vi "CreatePublicEvents.vi"(8 "error in (no error)":errorcluster, 11 "SMO":refnum<class "SMO.lvclass">) -> (0 "error out":errorcluster, 3 "SMO out":refnum<class "SMO.lvclass">)   [LabVIEW 2019, in "SMO.lvclass"]
doc: "JKI State Machine Objects (SMO) 1.3.0.56\nJKI - JKI\nCopyright (c) 2017, JKI"
uses:
  SMO.lvclass
  Typedefs/SMOState --Enum.ctl
  Typedefs/Reserve State--Enum.ctl
  SMO.lvclass/SMO.ctl
panel:
  # "For instructions on how to use the JKI State Machine Objects, examples and video tutorials, visit:\nhttp://jki.net/state-machine-objects/\n\nJKI State Machine Objects™\nhttp://jki.net/state-machine-objects/\nCopyright (C) 2005-2015, JKI <info@jki.net>\nALL RIGHTS RESERVED"
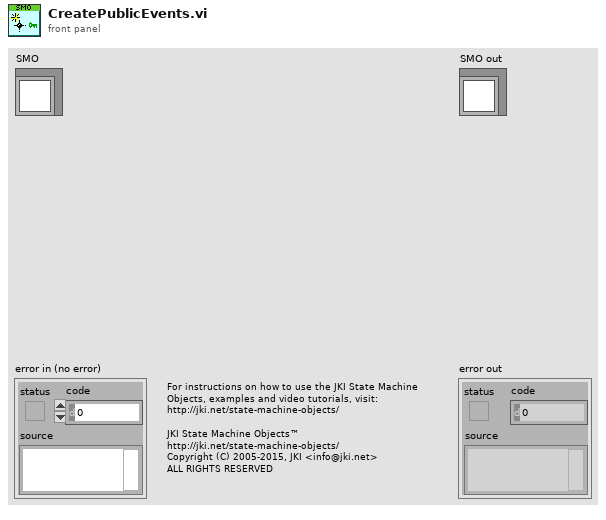
[diagram p1: front panel]
types:
  T1 = typedef "SMO.lvclass/Reserve State--Enum.ctl" = enum16{"Unreserved", "Reserved", "Self-locked"}
  T2 = typedef "SMO.lvclass/SMOState --Enum.ctl" = enum16{"unknown", "Created", "Started", "Stopped"}
  T3 = cluster{"error":refnum<user-event>, "SMO State":refnum<user-event>, "Reserve State":refnum<user-event>}
  T4 = typedef "SMO.lvclass/PrivateData--Ref.ctl" = refnum<data-value>
  T5 = typedef "SMO.lvclass/PrivateData--Cluster.ctl" = cluster{"Parent Call":T6, "Registered Processes":T7[], "Sync Notifier":refnum<notifier>, "Process Error Notifier":refnum<notifier>, "Protected Events":T8, "Public Events":T9, "SMO State":T2, "[Dependencies]":T10[], "[Attributes]":refnum<class "Attribute.lvclass">[], "Launcher Close":refnum<notifier>, "Caller Watchdog":refnum<queue>, "Accessibility":T11, "NbStaticDependencies":u32}
  T6 = typedef "SMO.lvclass/Parent Call--Enum.ctl" = enum16{"Allows parent to run", "Does not request parent to run"}
  T7 = typedef "SMO.lvclass/RegisteredProcessData--Cluster.ctl" = cluster{"Name":string, "Static VI Ref":refnum<vi>, "Running":bool, "NotifierRef":u32}
  T8 = typedef "SMO.lvclass/Protected Events.ctl" = cluster{"StopProcesses":refnum<user-event>, "AbortProcesses":refnum<user-event>, "Config Changed":refnum<user-event>, "Dependency":refnum<user-event>}
  T9 = typedef "SMO.lvclass/Public Events.ctl" = cluster{"Error":refnum<user-event>, "State":refnum<user-event>, "Reserve State":refnum<user-event>}
  T10 = typedef "SMO.lvclass/SMO Dependency--Cluster.ctl" = cluster{"Dependency":refnum<class "SMO.lvclass">, "Level":string}
  T11 = typedef "SMO.lvclass/Accessibility--Cluster.ctl" = cluster{"Lock Key":string, "Reserve State":T1}
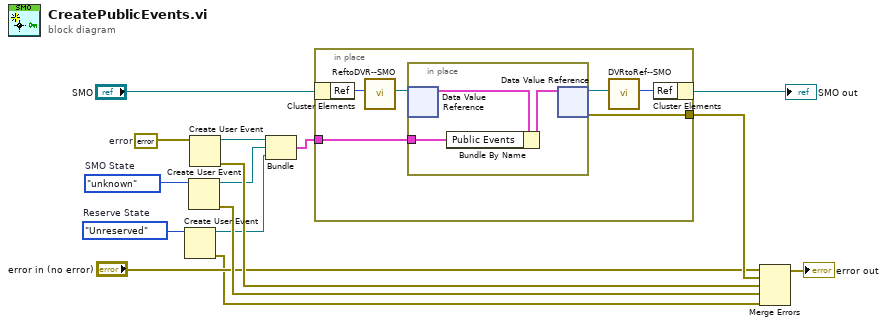
[diagram p0: block diagram]
diagram:
  w2 = Reserve_State--Enum."Unreserved"  # Reserve State
  w7 = SMOState_--Enum."unknown"  # SMO State
  w9 = errorcluster {"status"=FALSE, "code"=0, "source"=""}  # error
  n1 = Create User Event(user event datatype=w2) -> (user event=w1:refnum<user-event>, error out=w3:errorcluster)  [unwired: 1 in]
  n2 = Create User Event(user event datatype=w7) -> (user event=w6:refnum<user-event>, error out=w5:errorcluster)  [unwired: 1 in]
  n3 = Create User Event(user event datatype=w9) -> (user event=w10:refnum<user-event>, error out=w8:errorcluster)  [unwired: 1 in]
  n4 = Bundle("error"=w10, "SMO State"=w6, "Reserve State"=w1) -> (w11:T3)  [unwired: 1 in]
  n5 = in-place {
    in-place-border: w11 -> [w21]
    in-place-border: [w20] -> w12
    n6 = in-place-cluster #1("SMO") -> ("Ref"=w19:u32)
    n7 = call "ReftoDVR--SMO.vi"("Ref"=w19) -> ("Ref"=w18:T4)  [unwired: 10 in]
    n8 = in-place {
      in-place-border: w21 -> [w22]
      n9 = in-place-dvr #2(w18) -> (w24:T5)  [unwired: 1 out]
      n10 = Bundle By Name(cluster=w24, "Public Events"=w22) -> (w23:T5)
      n11 = in-place-dvr #2(w23) -> (w17:T4, w20:errorcluster)
    }
    n12 = call "DVRtoRef--SMO.vi"("Ref"=w17) -> ("Ref"=w16:u32)  [unwired: 10 in]
    n13 = in-place-cluster #1("Ref"=w16) -> (→"SMO out":refnum<class "SMO.lvclass">)
  }
  n14 = Merge Errors("error in (no error)", w12, w8, w5, w3) -> (→"error out":errorcluster)
